vi "GetVelocity.vi"(8 "error in (no error)":errorcluster, 11 "XYStage":refnum<class "XYStage.lvclass">) -> (0 "error out":errorcluster, 1 "Velocity (counts/s)":i32, 2 "Velocity (unit/s)":dbl, 3 "XYStage out":refnum<class "XYStage.lvclass">)   [LabVIEW 2013, in "XYStage.lvclass"]
doc: "---------------------------------------------------------------\nJKI State Machine Objects™\nhttp://jki.net/state-machine-objects/\nCopyright (C) 2005-2015, JKI <info@jki.net>\nALL RIGHTS RESERVEDJKI State Machine Objects (SMO) 1.0.0.4\nJKI - JKI\nCopyright (c) 2015, JKI"
uses:
  XYStage.lvclass
panel:
  # "For instructions on how to use the JKI State Machine Objects, examples and video tutorials, visit:\nhttp://jki.net/state-machine-objects/\n\nJKI State Machine Objects™\nhttp://jki.net/state-machine-objects/\nCopyright (C) 2005-2015, JKI <info@jki.net>\nALL RIGHTS RESERVED"
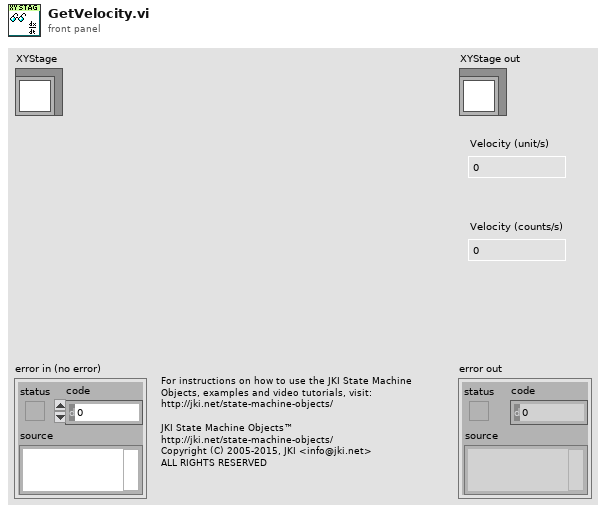
[diagram p1: front panel]
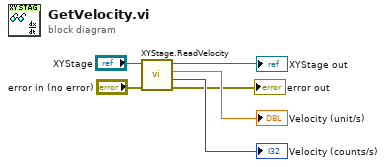
[diagram p0: block diagram]
diagram:
  n1 = call-dynamic "XYStage.ReadVelocity.vi"("error in (no error)"="error in (no error)", "XYStage in"="XYStage") -> ("error out"=→"error out":errorcluster, "Velocity (counts/s)"=→"Velocity (counts/s)":i32, "Velocity (units/s)"=→"Velocity (unit/s)":dbl, "XYStage out"=→"XYStage out":refnum<class "XYStage.lvclass">)  [unwired: 6 in]
